vi "EX3 6 12 1000.vi"() -> ()   [LabVIEW 2019]
panel:
  out "1000 !":dbl
  out "12!":dbl
  out "6!":i32
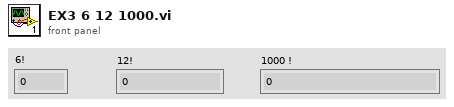
[diagram p1: front panel]
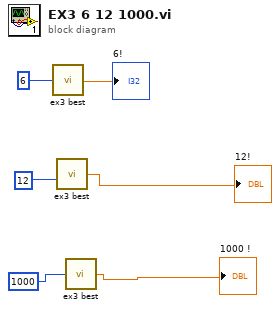
[diagram p0: block diagram]
diagram:
  n1 = call "ex3 best.vi"("Numeric 2"=6 ("N")) -> ("Numeric"=→"6!":dbl)
  n2 = call "ex3 best.vi"("Numeric 2"=12) -> ("Numeric"=→"12!":dbl)
  n3 = call "ex3 best.vi"("Numeric 2"=1000) -> ("Numeric"=→"1000 !":dbl)
